vi "Correctness Calculations.vi"(8 "Accepted":dbl, 11 "Measured":dbl) -> (3 "Error":dbl)   [LabVIEW 2014]
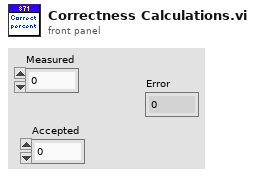
[diagram p1: front panel]
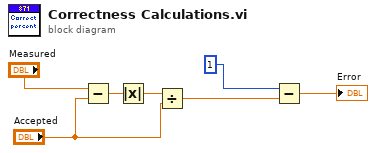
[diagram p0: block diagram]
diagram:
  n1 = Subtract(x="Measured", y="Accepted") -> (x-y=w6:dbl)
  n2 = Absolute Value(x=w6) -> (abs(x)=w5:dbl)
  n3 = Divide(x=w5, y="Accepted") -> (x/y=w3:dbl)
  n4 = Subtract(x=1, y=w3) -> (x-y=→"Error":dbl)
